vi "Main Control lasers.vi"() -> ()   [LabVIEW 2020]
uses:
  Control 1.ctl
  Control_states.ctl
  <vilib>/Analysis/baseanly.llb/Mean (DBL).vi
  <vilib>/ULx/Create Channel.llb/ULx Create Channel (AO-Voltage-Basic).vi
  <vilib>/ULx/Write.llb/ULx Write (Analog 1D DBL 1Chan NSamp).vi
  Global 1.vi
  <vilib>/ULx/Create Channel.llb/ULx Create Channel (DO-Digital Output).vi
  <vilib>/ULx/Write.llb/ULx Write (Digital Bool 1Line 1Point).vi
  <vilib>/ULx/Create Channel.llb/ULx Create Channel (AI-Voltage-Basic).vi
  <vilib>/ULx/Write.llb/ULx Write (Analog 1D DBL 1Chan 1Samp).vi
  <vilib>/ULx/Read.llb/ULx Read (Analog DBL 1Chan 1Samp).vi
  <vilib>/Analysis/NI_AALBase.lvlib
panel:
  in  "Tab Control 2":enum32{"Indicator"}(tab)
  out "Low Gain":dbl(graph)=1.648150384426117
  out "High Gain":dbl(graph)=143.05335879325867
  out "Data HG (mV)":dbl=143.05335879325867 format="%0.2f"
  out "Data LG (mV)":dbl=1.648150384426117 format="%0.2f"
  in  "SAVE":bool
  in  "stop":bool
  in  "Tab Control":T1(tab)
  in  "Frequency Selector (GHz)":i32(knob)=200 min=100 max=600 step=10 scale=100.0..600.0
  in  "Light":bool
  out "Stable output frequency":bool=TRUE
  in  "Stop Button":bool
  out "Current frequency (GHz)":dbl=200.0
  in  "Safety Switch":bool
  in  "Bias":bool
  in  "Sweep Activation":bool
  in  "Start (GHz)":dbl=100.0 min=100.0 max=600.0 step=10.0
  in  "Stop (GHz)":dbl=200.0 min=100.0 max=600.0 step=10.0
  in  "Time elapsed":T2
  in  "Time per point (ms)":u32=1000
  out "Current frequency monitor":dbl=200.0
  out "L2 ini":dbl=1.0008
  out "L1 ini":dbl=0.62712
  in  "contador":dbl=40.0
  in  "LD1 laser point":dbl=0.62712
  out "Current laser 1 (mA)":dbl=156.78
  out "Current laser 2 (mA)":dbl=250.2
  out "Laser":dbl=3.0
  out "String":string="estoy aqui"
  out "Signal OFF LG":dbl=-0.0037846416234970093 format="%0.2f"
  out "Signal ON LG":dbl=-0.005738005042076111 format="%0.2f"
  out "Difference LG":dbl=1.9533634185791016
  out "Difference HG":dbl=134.41584110259976
  out "Signal OFF HG":dbl=-3.054205846786499 format="%0.2f"
  out "Signal ON HG":dbl=-3.188621687889099 format="%0.2f"
  in  "Integration time (ms)":i32=20
  out "x+y":dbl=40.0
  in  "Ring":u16(ring) items=["600,93", "590,96", "580,92", "570,94", "561", "550,96", "541", "530,9", "520,97", "510,98", "500,96", "490,89", "480,99", "470,91", "460,92", "450,98", "440,98", "430,96", "420,95", "410,99", "400,92", "390,92", "381", "370,99", "360,92", "350,91", "340,97", "330,95", "320,99", "310,94", "300,94", "290,85", "280,97", "270,99", "260,9", "250,89", "240,92", "230,87", "220,83", "210,92", "200,98", "190,88", "180,96", "170,96", "160,95", "150,82", "140,96", "130,89", "120,87", "110,9", "100,95", "91", "80,85", "70,91", "60,99", "50,8", "40,88", "30,84", "20,78", "10,7"]
  out "OldVal":dbl
  out "corriente L1 2":dbl
  out "ok":bool
  in  "LD2 laser point":dbl=1.0008
  # "ON Sequence"
  # "OFF Sequence"
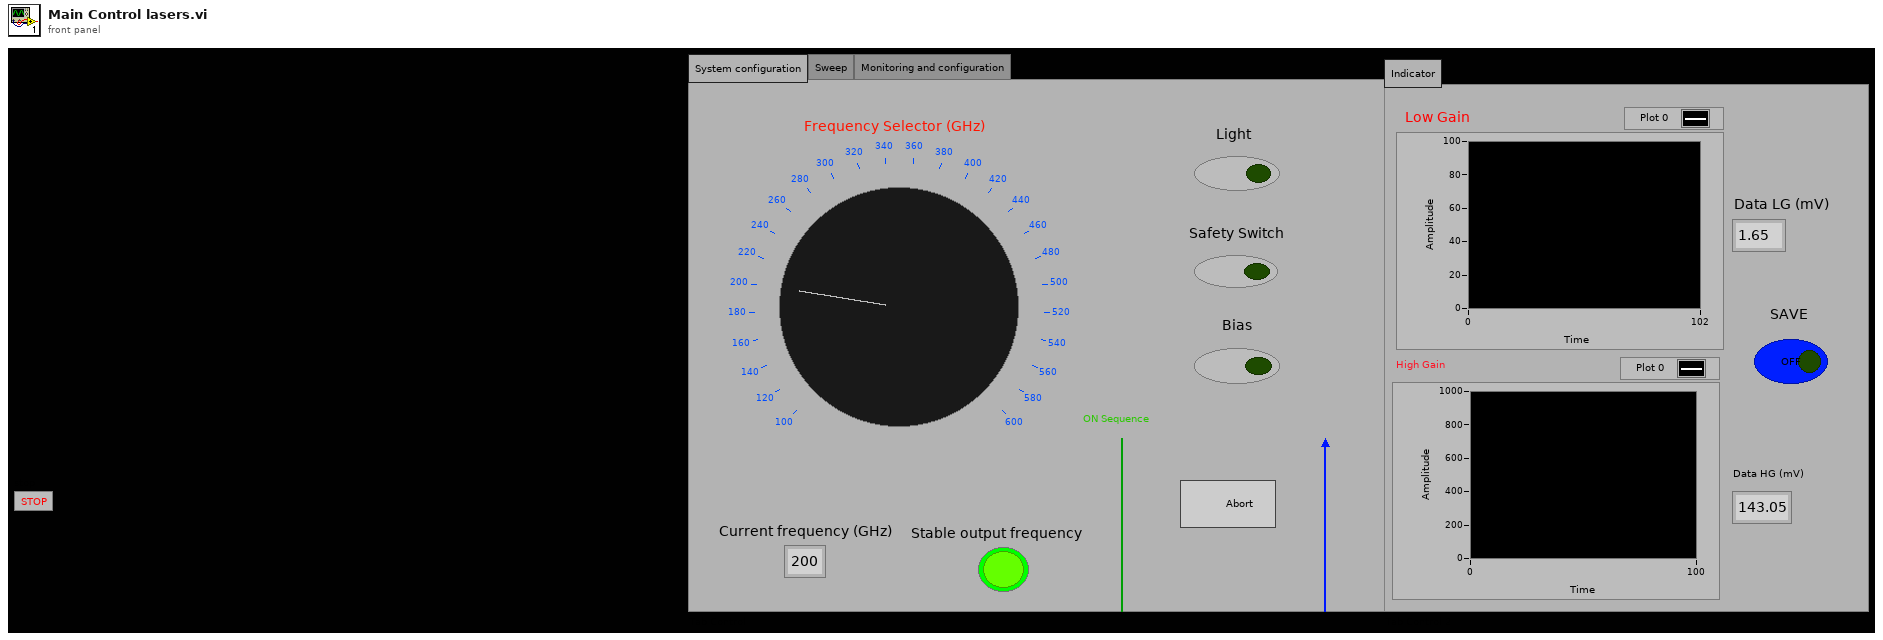
[diagram p1: front panel]
types:
  T1 = enum32{"System configuration", "Sweep", "Monitoring and configuration"}
  T2 = typedef "Control 1.ctl" = dbl
  T3 = typedef "Control_states.ctl" = enum16{"Rele", "Enable", "Corriente L2", "Sweep", "Atenuador", "Initializing", "Setting", "Modulacion", "Saving", "Control", "Closing"}
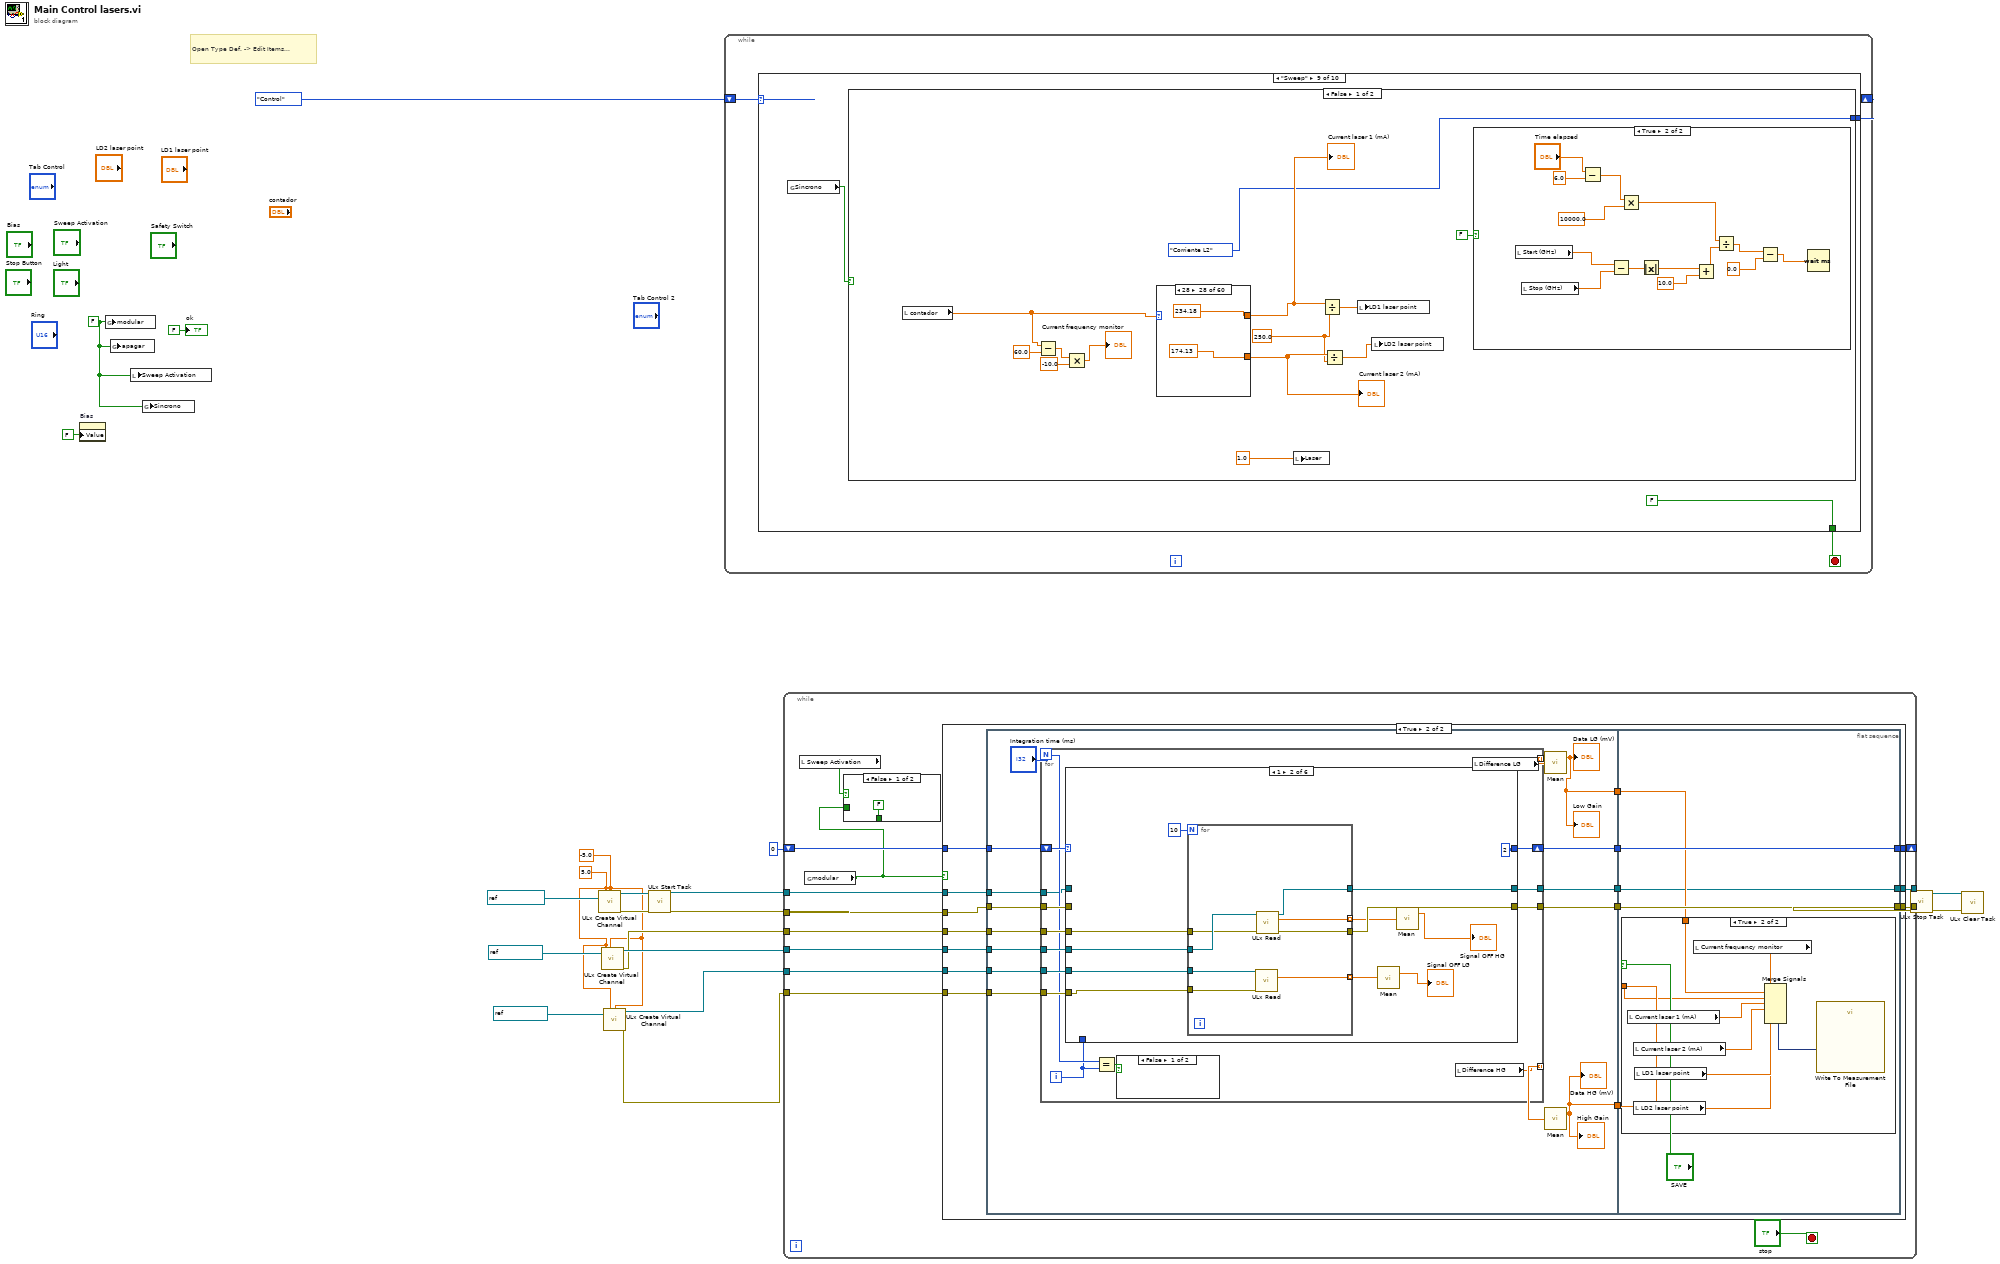
[diagram p0: block diagram]
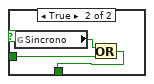
[diagram p2: hidden frame]
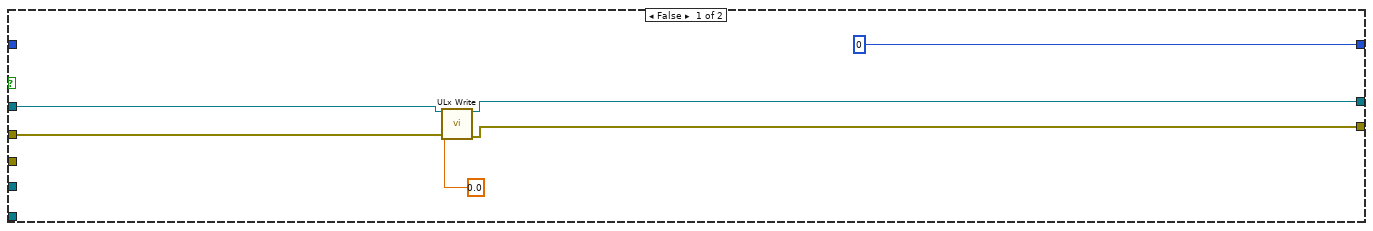
[diagram p3: hidden frame]
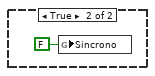
[diagram p4: hidden frame]
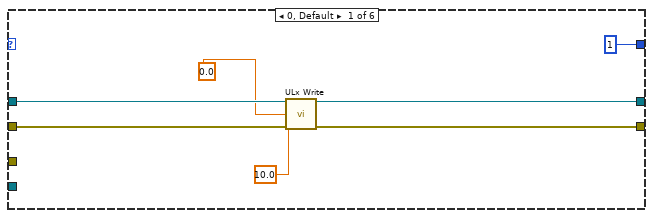
[diagram p5: hidden frame]
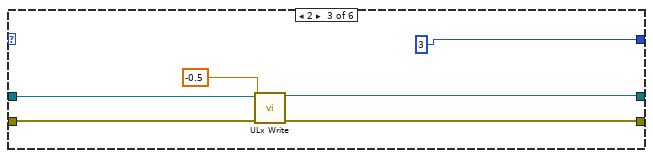
[diagram p6: hidden frame]
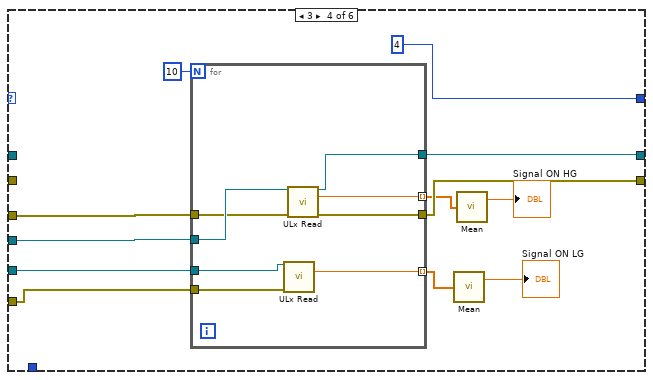
[diagram p7: hidden frame]
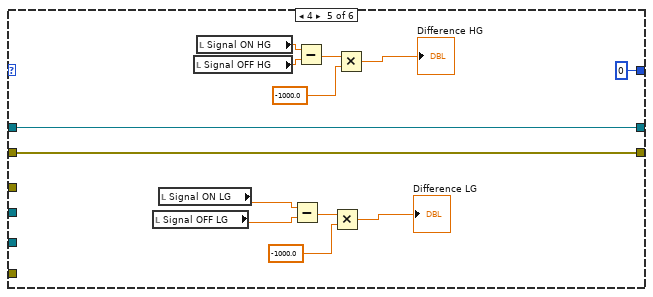
[diagram p8: hidden frame]
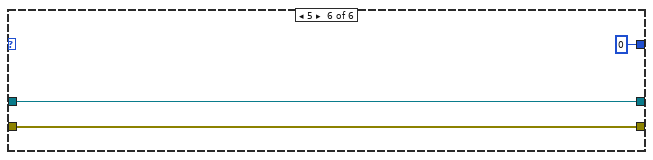
[diagram p9: hidden frame]
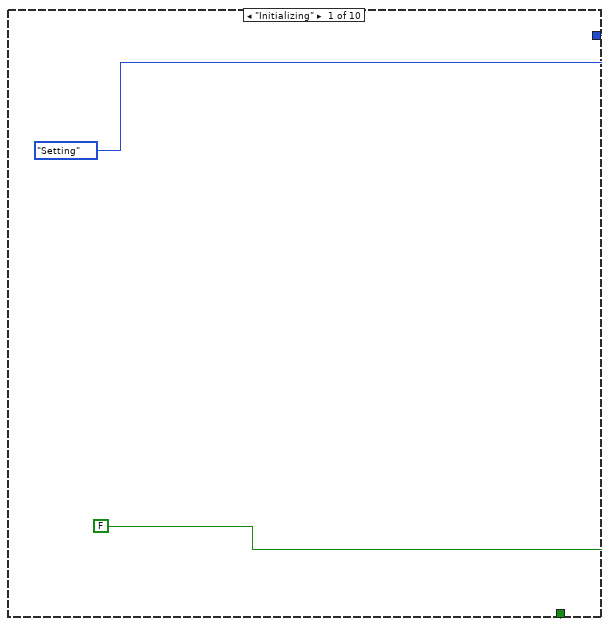
[diagram p11: hidden frame]
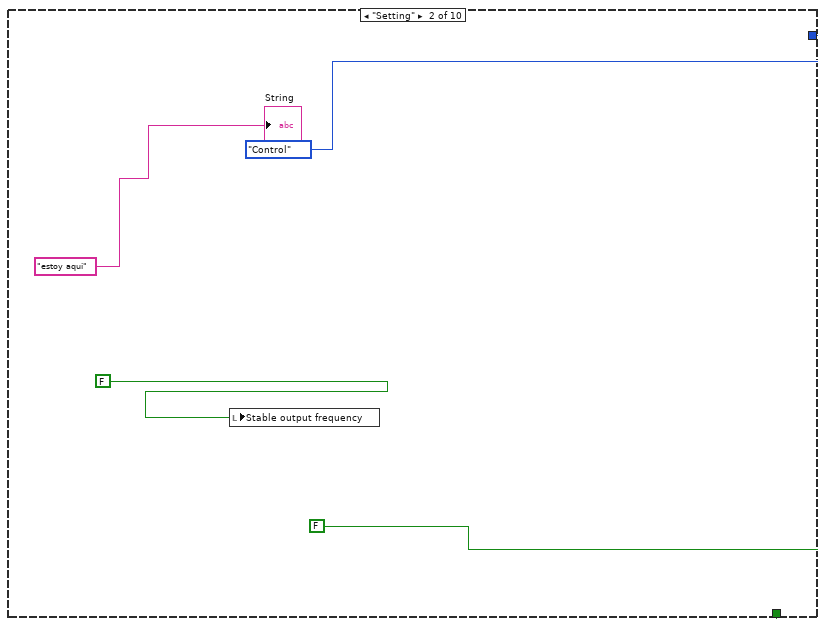
[diagram p12: hidden frame]
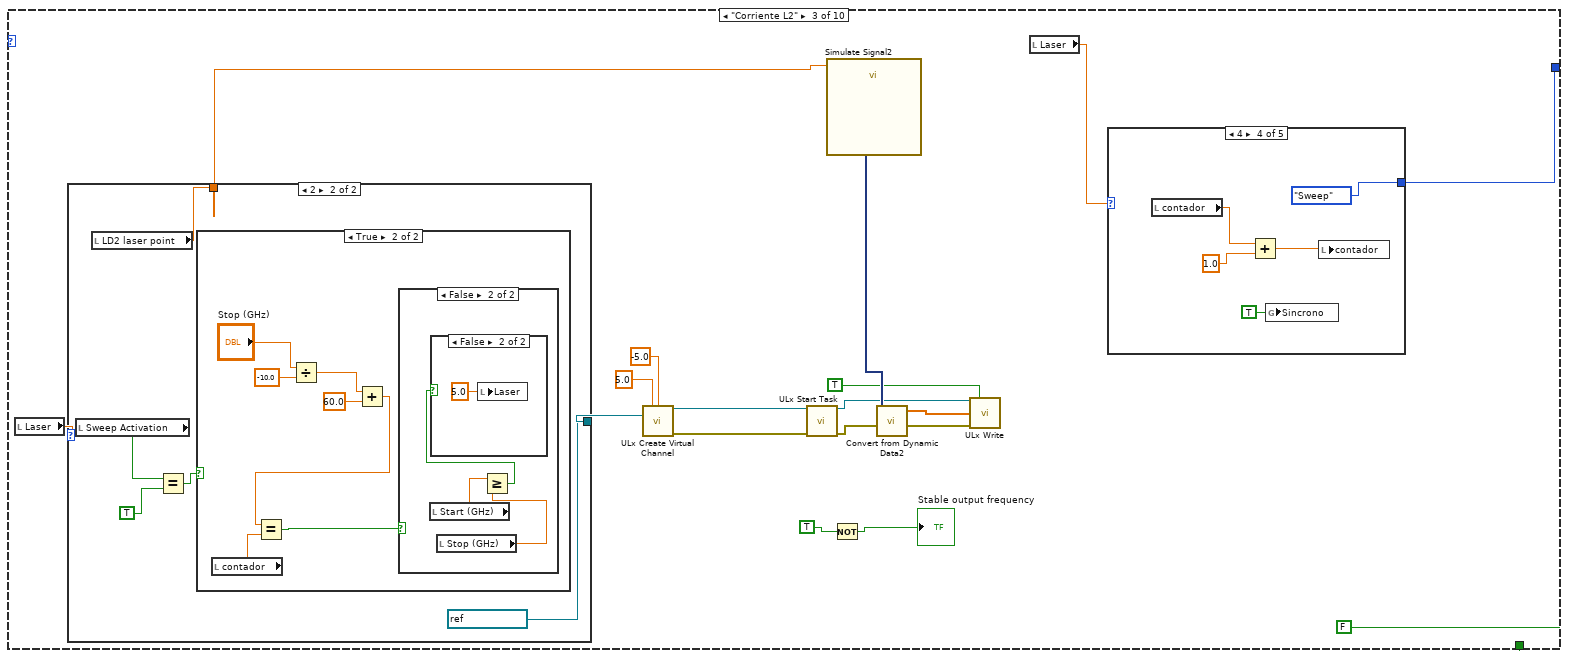
[diagram p13: hidden frame]
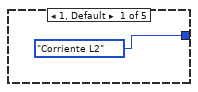
[diagram p14: hidden frame]
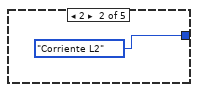
[diagram p15: hidden frame]
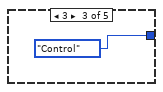
[diagram p16: hidden frame]
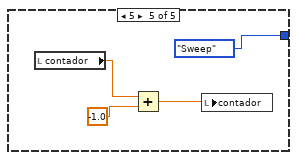
[diagram p17: hidden frame]
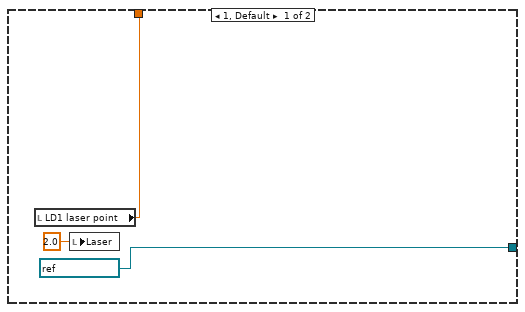
[diagram p18: hidden frame]
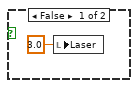
[diagram p19: hidden frame]
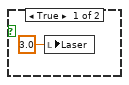
[diagram p20: hidden frame]
diagram:
  w2 = -5.0 ("minimum value")
  w3 = 5.0 ("maximum value")
  w6 = FALSE ("modular")
  # "Open Type Def. -> Edit Items..."
  n1 = property on="Bias" class="Bool (strict)"("Value"=FALSE ("Modular")) -> ()  [unwired: 2 in, 2 out]
  n2 = global write "Global 1.vi" "modular"(w6) -> ()
  n3 = global write "Global 1.vi" "apagar"(w6) -> ()
  n4 = local write "Sweep Activation"(w6) -> ()
  n5 = global write "Global 1.vi" "Sincrono"(w6) -> ()
  n6 = call-poly <vilib>:"ULx Create Virtual Channel.vi"("maximum value"=w3, "minimum value"=w2, "physical channels"=refnum<k21> "Dev0/Ao3") -> ("task out"=w19:refnum<k24>, "error out"=w18:errorcluster)  [unwired: 11 in]
  n7 = call-poly <vilib>:"ULx Create Virtual Channel.vi"("maximum value"=w3, "minimum value"=w2, "physical channels"=refnum<k21> "Dev0/Ai0") -> ("task out"=w12:refnum<k24>, "error out"=w11:errorcluster)  [unwired: 11 in]
  n8 = call-poly <vilib>:"ULx Create Virtual Channel.vi"("maximum value"=w3, "minimum value"=w2, "physical channels"=refnum<k21> "Dev0/Ai1") -> ("task out"=w1:refnum<k24>, "error out"=w4:errorcluster)  [unwired: 11 in]
  n9 = call <vilib>:"ULx Start Task.vi"("task in"=w19, "error in"=w18) -> ("task out"=w16:refnum<k24>, "error out"=w15:errorcluster)  [unwired: 12 in]
  n10 = while {
    shift-right: [w23] -> _
    shift-left: Control_states."Control" -> [w25]
    stop <- w24 stop-if-true
    n11 = case shown="\"Sweep\"" w25 {
      tunnel: [FALSE FALSE FALSE FALSE FALSE w87 FALSE FALSE FALSE FALSE] -> w24
      tunnel: [Control_states."Setting" Control_states."Control" w37 Control_states."Saving" Control_states."Control" Control_states."Closing" Control_states."Control" w99 w261 Control_states."Control"] -> w23
      frame "Initializing" {
      }
      frame "Setting" {
        n12 = local write "Stable output frequency"(FALSE ("L1 ok")) -> ()
        "String" <- "estoy aqui"
      }
      frame "Corriente L2" {
        n13 = local read "Laser"() -> (w39:dbl)
        n14 = case shown="2" w39 {
          tunnel: [refnum<k21> "Dev0/Ao0" ("physical channels") refnum<k21> "Dev0/Ao1" ("physical channels")] -> w46
          tunnel: [w62 w67] -> w38
          frame 1, Default {
            n15 = local read "LD1 laser point"() -> (w62:dbl)
            n16 = local write "Laser"(2.0 ("Laser")) -> ()
          }
          frame 2 {
            n17 = local read "Sweep Activation"() -> (w64:bool)
            n18 = local read "LD2 laser point"() -> (w67:dbl)
            n19 = Equal?(x=w64, y=TRUE) -> (x = y?=w66:bool)
            n20 = case shown="True" w66 {
              frame False {
                n21 = local write "Laser"(3.0 ("Laser")) -> ()
              }
              frame True {
                n22 = local read "contador"() -> (w75:dbl)
                n23 = Divide(x="Stop (GHz)", y=-10.0) -> (x/y=w73:dbl)
                n24 = Add(x=w73, y=60.0) -> (x+y=w70:dbl)
                n25 = Equal?(x=w70, y=w75) -> (x = y?=w76:bool)
                n26 = case shown="False" w76 {
                  frame True {
                    n27 = local write "Laser"(3.0 ("Laser")) -> ()
                  }
                  frame False {
                    n28 = local read "Start (GHz)"() -> (w80:dbl)
                    n29 = local read "Stop (GHz)"() -> (w79:dbl)
                    n30 = Greater Or Equal?(x=w80, y=w79) -> (x >= y?=w78:bool)
                    n31 = case shown="False" w78 {
                      frame True {
                        n32 = local write "Laser"(4.0 ("Laser")) -> ()
                      }
                      frame False {
                        n33 = local write "Laser"(5.0 ("Laser")) -> ()
                      }
                    }
                  }
                }
              }
            }
          }
        }
        n34 = call-poly <vilib>:"ULx Create Virtual Channel.vi"("maximum value"=5.0, "minimum value"=-5.0, "physical channels"=w46) -> ("task out"=w47:refnum<k24>, "error out"=w48:errorcluster)  [unwired: 11 in]
        n35 = call <vilib>:"ULx Start Task.vi"("task in"=w47, "error in"=w48) -> ("task out"=w42:refnum<k24>, "error out"=w41:errorcluster)  [unwired: 12 in]
        n36 = call "Simulate Signal2"("Offset"=w38) -> ("DC"=w45:dynamicdata)  [unwired: 13 in, 1 out]
        n37 = Not(x=TRUE) -> (.not. x?=→"Stable output frequency":bool)
        n38 = call "Convert from Dynamic Data2"("Dynamic Data Type"=w45) -> ("Array"=w44:dbl[])  [unwired: 3 in]
        n39 = call-poly <vilib>:"ULx Write.vi"("task in"=w42, "auto start"=TRUE, "data"=w44, "error in"=w41) -> ()  [unwired: 9 in, 3 out]
        n40 = local read "Laser"() -> (w36:dbl)
        n41 = case shown="4" w36 {
          tunnel: [Control_states."Corriente L2" Control_states."Corriente L2" Control_states."Control" Control_states."Sweep" Control_states."Sweep"] -> w37
          frame 1, Default {
          }
          frame 2 {
          }
          frame 3 {
          }
          frame 4 {
            n42 = local read "contador"() -> (w55:dbl)
            n43 = Add(x=w55, y=1.0) -> (x+y=w54:dbl)
            n44 = global write "Global 1.vi" "Sincrono"(TRUE ("Sincrono")) -> ()
            n45 = local write "contador"(w54) -> ()
          }
          frame 5 {
            n46 = local read "contador"() -> (w59:dbl)
            n47 = Add(x=w59, y=-1.0) -> (x+y=w58:dbl)
            n48 = local write "contador"(w58) -> ()
          }
        }
      }
      frame "Modulacion" {
      }
      frame "Saving" {
      }
      frame "Closing" {
        w87 = TRUE
        n49 = local write "Stable output frequency"(TRUE ("L1 ok")) -> ()
        n50 = global write "Global 1.vi" "apagar"(w87) -> ()
      }
      frame "Rele" {
        n51 = call-poly <vilib>:"ULx Create Virtual Channel.vi"("lines"=refnum<k21> "Dev0/AuxPort/Do9") -> ("task out"=w94:refnum<k24>, "error out"=w93:errorcluster)  [unwired: 13 in]
        n52 = local read "Safety Switch"() -> (w90:bool)
        n53 = call <vilib>:"ULx Start Task.vi"("task in"=w94, "error in"=w93) -> ("task out"=w92:refnum<k24>, "error out"=w91:errorcluster)  [unwired: 12 in]
        n54 = call-poly <vilib>:"ULx Write.vi"("task in"=w92, "data"=w90, "error in"=w91) -> ()  [unwired: 10 in, 3 out]
      }
      frame "Control", Default {
        n55 = event shown="[3] \"Frequency Selector (GHz)\": Value Change" {
          selector: _ -> [_ _ _ _ _ _ _ _]
          dyn-events: _ -> [_ _ _ _ _ _ _ _]
          timeout: 1 -> [_ _ _ _ _ _ _ _]
          tunnel: [Control_states."Control" Control_states."Atenuador" _ Control_states."Corriente L2" Control_states."Sweep" Control_states."Closing" Control_states."Enable" Control_states."Rele"] -> w99
          event Timeout {
            n56 = event-data() -> ()  [unwired: 1 in, 3 out]
            n57 = local read "LD2 laser point"() -> (→"L2 ini":dbl)
            n58 = local read "LD1 laser point"() -> (→"L1 ini":dbl)
            n59 = local write "Stable output frequency"(TRUE ("ok")) -> ()
          }
          event "LD1 laser point", "LD2 laser point": Value Change {
            n60 = event-data() -> ("OldVal"=w112:dbl)  [unwired: 1 in, 5 out]
            "OldVal" <- w112
            n61 = local read "LD1 laser point"() -> (w109:dbl)
            n62 = local read "L1 ini"() -> (w110:dbl)
            "corriente L1 2" <- w110
            n63 = Not Equal?(x=w110, y=w109) -> (x != y?=w108:bool)
            n64 = Equal?(x=w110, y=w112) -> (x = y?=w107:bool)
            n65 = And(x=w107, y=w108) -> (x .and. y?=w106:bool)
            n66 = case shown="False" w106 {
              tunnel: [2.0 ("Laser") 1.0 ("Laser")] -> w111
              frame False {
              }
              frame True {
              }
            }
            "Laser" <- w111
          }
          event "Bias": Value Change {
            n67 = event-data() -> ()  [unwired: 1 in, 6 out]
            n68 = global read "Global 1.vi" "modular"() -> (w116:bool)
            n69 = Not(x=w116) -> (.not. x?=w115:bool)
            n70 = global write "Global 1.vi" "modular"(w115) -> ()
          }
          event "Frequency Selector (GHz)": Value Change {
            w120 = 250.0 ("y")
            n71 = event-data() -> ()  [unwired: 1 in, 6 out]
            n72 = Divide(x="Frequency Selector (GHz)", y=-10.0) -> (x/y=w126:dbl)
            n73 = Add(x=w126, y=60.0) -> (x+y=w122:dbl)
            "x+y" <- w122
            n74 = case shown="9" w122 {
              tunnel: [52.69 57.03 59.36 63.7 66.7 69.7 73.37 76.71 82.05 86.05 90.39 94.39 97.73 102.4 107.07 112.07 116.08 121.42 126.75 131.43 136.1 141.77 146.77 152.11 157.45 162.79 168.46 174.13 180.13 186.14 192.48 198.48 204.16 210.83 216.83 223.51 229.85 236.85 243.19 250.2 257.54 264.21 271.55 278.56 286.23 293.57 300.91 308.58 316.26 323.93 331.94 339.94 347.95 355.96 364.3 372.31 380.65 388.99 397.33 46.68] -> w119
              tunnel: [398.66 392.99 386.98 381.31 375.31 369.3 363.3 357.29 351.62 345.61 339.61 333.6 327.27 321.26 315.25 309.25 302.91 296.91 290.9 284.56 278.22 272.22 265.88 259.54 253.2 246.86 240.52 234.18 227.84 221.5 215.17 208.83 202.15 195.82 189.14 182.8 176.13 169.79 163.12 156.78 150.44 143.77 137.43 130.76 124.42 118.08 111.41 105.07 98.73 92.39 86.39 80.05 74.04 68.04 62.03 56.02 50.35 44.68 39.01 404] -> w117
              frame 1, Default {
              }
              frame 2 {
              }
              frame 3 {
              }
              frame 4 {
              }
              frame 5 {
              }
              frame 6 {
              }
              frame 7 {
              }
              frame 8 {
              }
              frame 9 {
              }
              frame 10 {
              }
              frame 11 {
              }
              frame 12 {
              }
              frame 13 {
              }
              frame 14 {
              }
              frame 15 {
              }
              frame 16 {
              }
              frame 17 {
              }
              frame 18 {
              }
              frame 19 {
              }
              frame 20 {
              }
              frame 21 {
              }
              frame 22 {
              }
              frame 23 {
              }
              frame 24 {
              }
              frame 25 {
              }
              frame 26 {
              }
              frame 27 {
              }
              frame 28 {
              }
              frame 29 {
              }
              frame 30 {
              }
              frame 31 {
              }
              frame 32 {
              }
              frame 33 {
              }
              frame 34 {
              }
              frame 35 {
              }
              frame 36 {
              }
              frame 37 {
              }
              frame 38 {
              }
              frame 39 {
              }
              frame 40 {
              }
              frame 41 {
              }
              frame 42 {
              }
              frame 43 {
              }
              frame 44 {
              }
              frame 45 {
              }
              frame 46 {
              }
              frame 47 {
              }
              frame 48 {
              }
              frame 49 {
              }
              frame 50 {
              }
              frame 51 {
              }
              frame 52 {
              }
              frame 53 {
              }
              frame 54 {
              }
              frame 55 {
              }
              frame 56 {
              }
              frame 57 {
              }
              frame 58 {
              }
              frame 59 {
              }
              frame 0 {
              }
            }
            n75 = Divide(x=w117, y=w120) -> (x/y=w123:dbl)
            n76 = Divide(x=w119, y=w120) -> (x/y=w124:dbl)
            n77 = local write "Laser"(1.0 ("Laser")) -> ()
            n78 = local write "LD1 laser point"(w123) -> ()
            n79 = local write "LD2 laser point"(w124) -> ()
            "Current frequency (GHz)" <- "Frequency Selector (GHz)"
          }
          event "Sweep Activation": Value Change {
            n80 = event-data() -> ()  [unwired: 1 in, 6 out]
            n81 = Divide(x="Start (GHz)", y=-10.0) -> (x/y=w251:dbl)
            n82 = Add(x=w251, y=60.0) -> (x+y=w249:dbl)
            n83 = local write "contador"(w249) -> ()
          }
          event "Stop Button": Value Change {
            n84 = event-data() -> ()  [unwired: 1 in, 6 out]
            n85 = property on="Bias" class="Bool (strict)"("Value"=FALSE ("Modular")) -> ()  [unwired: 2 in, 2 out]
          }
          event "Light": Value Change {
            n86 = event-data() -> ()  [unwired: 1 in, 6 out]
          }
          event "Safety Switch": Value Change {
            n87 = event-data() -> ()  [unwired: 1 in, 6 out]
          }
        }
      }
      frame "Sweep" {
        n88 = global read "Global 1.vi" "Sincrono"() -> (w260:bool)
        n89 = case shown="False" w260 {
          tunnel: [Control_states."Corriente L2" Control_states."Control"] -> w261
          frame False {
            w269 = 250.0
            n90 = local read "contador"() -> (w265:dbl)
            n91 = Subtract(x=w265, y=60.0) -> (x-y=w264:dbl)
            n92 = Multiply(x=w264, y=-10.0) -> (x*y=→"Current frequency monitor":dbl)
            n93 = case shown="28" w265 {
              tunnel: [398.66 392.99 386.98 381.31 375.31 369.3 363.3 357.29 351.62 345.61 339.61 333.6 327.27 321.26 315.25 309.25 302.91 296.91 290.9 284.56 278.22 272.22 265.88 259.54 253.2 246.86 240.52 234.18 227.84 221.5 215.17 208.83 202.15 195.82 189.14 182.8 176.13 169.79 163.12 156.78 150.44 143.77 137.43 130.76 124.42 118.08 111.41 105.07 98.73 92.39 86.39 80.05 74.04 68.04 62.03 56.02 50.35 44.68 39.01 404.0] -> w271
              tunnel: [52.69 57.03 59.36 63.7 66.7 69.7 73.37 76.71 82.05 86.05 90.39 94.39 97.73 102.4 107.07 112.07 116.08 121.42 126.75 131.43 136.1 141.77 146.77 152.11 157.45 162.79 168.46 174.13 180.13 186.14 192.48 198.48 204.16 210.83 216.83 223.51 229.85 236.85 243.19 250.2 257.54 264.21 271.55 278.56 286.23 293.57 300.91 308.58 316.26 323.93 331.94 339.94 347.95 355.96 364.3 372.31 380.65 388.99 397.33 46.68] -> w272
              frame 1, Default {
              }
              frame 2 {
              }
              frame 3 {
              }
              frame 4 {
              }
              frame 5 {
              }
              frame 6 {
              }
              frame 7 {
              }
              frame 8 {
              }
              frame 9 {
              }
              frame 10 {
              }
              frame 11 {
              }
              frame 12 {
              }
              frame 13 {
              }
              frame 14 {
              }
              frame 15 {
              }
              frame 16 {
              }
              frame 17 {
              }
              frame 18 {
              }
              frame 19 {
              }
              frame 20 {
              }
              frame 21 {
              }
              frame 22 {
              }
              frame 23 {
              }
              frame 24 {
              }
              frame 25 {
              }
              frame 26 {
              }
              frame 27 {
              }
              frame 28 {
              }
              frame 29 {
              }
              frame 30 {
              }
              frame 31 {
              }
              frame 32 {
              }
              frame 33 {
              }
              frame 34 {
              }
              frame 35 {
              }
              frame 36 {
              }
              frame 37 {
              }
              frame 38 {
              }
              frame 39 {
              }
              frame 40 {
              }
              frame 41 {
              }
              frame 42 {
              }
              frame 43 {
              }
              frame 44 {
              }
              frame 45 {
              }
              frame 46 {
              }
              frame 47 {
              }
              frame 48 {
              }
              frame 49 {
              }
              frame 50 {
              }
              frame 51 {
              }
              frame 52 {
              }
              frame 53 {
              }
              frame 54 {
              }
              frame 55 {
              }
              frame 56 {
              }
              frame 57 {
              }
              frame 58 {
              }
              frame 59 {
              }
              frame 0 {
              }
            }
            "Current laser 1 (mA)" <- w271
            "Current laser 2 (mA)" <- w272
            n94 = local write "Laser"(1.0 ("Laser")) -> ()
            n95 = Divide(x=w271, y=w269) -> (x/y=w273:dbl)
            n96 = Divide(x=w272, y=w269) -> (x/y=w274:dbl)
            n97 = local write "LD1 laser point"(w273) -> ()
            n98 = local write "LD2 laser point"(w274) -> ()
            n99 = case shown="True" FALSE {
              frame False {
                n100 = Wait (ms)(milliseconds to wait="Time per point (ms)") -> ()  [unwired: 1 out]
              }
              frame True {
                n101 = local read "Start (GHz)"() -> (w279:dbl)
                n102 = local read "Stop (GHz)"() -> (w278:dbl)
                n103 = Subtract(x="Time elapsed", y=6.0) -> (x-y=w280:T2)
                n104 = Subtract(x=w279, y=w278) -> (x-y=w277:dbl)
                n105 = Multiply(x=w280, y=10000.0) -> (x*y=w289:T2)
                n106 = Absolute Value(x=w277) -> (abs(x)=w276:dbl)
                n107 = Add(x=w276, y=10.0) -> (x+y=w288:dbl)
                n108 = Divide(x=w289, y=w288) -> (x/y=w285:T2)
                n109 = Subtract(x=w285, y=0.0) -> (x-y=w284:T2)
                n110 = Wait (ms)(milliseconds to wait=w284) -> ()  [unwired: 1 out]
              }
            }
          }
          frame True {
          }
        }
      }
      frame "Enable" {
        n111 = call-poly <vilib>:"ULx Create Virtual Channel.vi"("lines"=refnum<k21> "Dev0/AuxPort/Do8") -> ("task out"=w416:refnum<k24>, "error out"=w417:errorcluster)  [unwired: 13 in]
        n112 = call <vilib>:"ULx Start Task.vi"("task in"=w416, "error in"=w417) -> ("task out"=w414:refnum<k24>, "error out"=w413:errorcluster)  [unwired: 12 in]
        n113 = local read "Light"() -> (w411:bool)
        n114 = Not(x=w411) -> (.not. x?=w412:bool)
        n115 = call-poly <vilib>:"ULx Write.vi"("task in"=w414, "data"=w412, "error in"=w413) -> ()  [unwired: 10 in, 3 out]
        n116 = case shown="True" w411 {
          frame False {
          }
          frame True {
            w420 = 200 ("Value (Signaling)")
            n117 = local write "Current frequency (GHz)"(w420) -> ()
            n118 = property on="Frequency Selector (GHz)" class="Knob (strict)"("Val(Sgnl)"=w420) -> ()  [unwired: 2 in, 2 out]
          }
        }
      }
    }
  }
  n119 = while {
    tunnel: w16 -> [w433]
    tunnel: w15 -> [w432]
    shift-right: [w430] -> _
    shift-left: 0 -> [w431]
    tunnel: w12 -> [w429]
    tunnel: w11 -> [w428]
    tunnel: [w427] -> w10
    tunnel: [w426] -> w9
    tunnel: w1 -> [w423]
    tunnel: w4 -> [w422]
    stop <- "stop" stop-if-true
    n120 = local read "Sweep Activation"() -> (w424:bool)
    n121 = global read "Global 1.vi" "modular"() -> (w421:bool)
    n122 = case shown="False" w424 {
      tunnel: w421 -> [_ w436]
      tunnel: [FALSE w435] -> _
      frame False {
      }
      frame True {
        n123 = global read "Global 1.vi" "Sincrono"() -> (w437:bool)
        n124 = Or(x=w437, y=w436) -> (x .or. y?=w435:bool)
      }
    }
    n125 = case shown="True" w421 {
      tunnel: w433 -> [w442 w450]
      tunnel: w432 -> [w441 w458]
      tunnel: w431 -> [_ w457]
      tunnel: [0 w456] -> w430
      tunnel: w429 -> [_ w455]
      tunnel: w428 -> [_ w454]
      tunnel: [w440 w449] -> w427
      tunnel: [w439 w453] -> w426
      tunnel: w423 -> [_ w452]
      tunnel: w422 -> [_ w451]
      frame False {
        n126 = call-poly <vilib>:"ULx Write.vi"("task in"=w442, "data"=0.0, "error in"=w441) -> ("task out"=w440:refnum<k24>, "error out"=w439:errorcluster)  [unwired: 10 in, 1 out]
      }
      frame True {
        n127 = flat-sequence {
          tunnel: w458 -> [w473]
          tunnel: w457 -> [w472]
          tunnel: w455 -> [w470]
          tunnel: w454 -> [w469]
          tunnel: w452 -> [w466]
          tunnel: w451 -> [w465]
          tunnel: w450 -> [w463]
          tunnel: [w471] -> w448
          tunnel: [w468] -> w447
          tunnel: [w462] -> w446
          tunnel: [w460] -> w445
          tunnel: [w459] -> w444
          tunnel: [w559] -> w449
          tunnel: [w563] -> w453
          tunnel: [w564] -> w456
          tunnel: w448 -> [w564]
          tunnel: w447 -> [w563]
          tunnel: w446 -> [w559]
          tunnel: w445 -> [w561]
          tunnel: w444 -> [w560]
          frame #0 {
            n128 = for {
              N: "Integration time (ms)" -> [w479]
              tunnel: w470 -> [w485]
              tunnel: w469 -> [w484]
              shift-right: [w486] -> w471
              shift-left: w472 -> [w487]
              tunnel: [w475] -> w464 mode=indexing
              tunnel: w466 -> [w481]
              tunnel: w465 -> [w480]
              tunnel: [w474] -> w461 mode=indexing
              tunnel: w463 -> [w478]
              tunnel: w473 -> [w488]
              tunnel: [w483] -> w468
              tunnel: [w477] -> w462
              i -> [w476]
              n129 = case shown="1" w487 {
                tunnel: w478 -> [w496 _ w522 _ w544 w557]
                tunnel: w488 -> [w495 _ w521 _ w543 w556]
                tunnel: [w493 w504 w520 w531 w544 w557] -> w477
                tunnel: [w492 w503 w519 w530 w543 w556] -> w483
                tunnel: [1 2 3 4 0 0] -> w486
                tunnel: w485 -> [_ w508 _ w532 _ _]
                tunnel: w484 -> [_ w507 _ w533 _ _]
                tunnel: w481 -> [_ w500 _ w526 _ _]
                tunnel: w480 -> [_ w499 _ w525 _ _]
                tunnel: w476 -> [_ _ _ _ _ _]
                frame 0, Default {
                  n130 = call-poly <vilib>:"ULx Write.vi"("task in"=w496, "data"=0.0 ("Min modulación"), "timeout"=10.0, "error in"=w495) -> ("task out"=w493:refnum<k24>, "error out"=w492:errorcluster)  [unwired: 9 in, 1 out]
                }
                frame 1 {
                  n131 = for {
                    N: 10 -> [_]
                    tunnel: w508 -> [w516]
                    tunnel: w507 -> [w515]
                    tunnel: [w514] -> w502 mode=indexing
                    tunnel: [w513] -> w504
                    tunnel: [w512] -> w503
                    tunnel: w500 -> [w511]
                    tunnel: w499 -> [w510]
                    tunnel: [w509] -> w498 mode=indexing
                    n132 = call-poly <vilib>:"ULx Read.vi"("task in"=w511, "error in"=w510) -> ("data"=w509:dbl)  [unwired: 11 in, 2 out]
                    n133 = call-poly <vilib>:"ULx Read.vi"("task in"=w516, "error in"=w515) -> ("task out"=w513:refnum<k24>, "data"=w514:dbl, "error out"=w512:errorcluster)  [unwired: 11 in]
                  }
                  n134 = call-poly <vilib>:"Mean.vi"("X"=w498) -> ("mean"=→"Signal OFF LG":dbl)  [unwired: 1 out]
                  n135 = call-poly <vilib>:"Mean.vi"("X"=w502) -> ("mean"=→"Signal OFF HG":dbl)  [unwired: 1 out]
                }
                frame 2 {
                  n136 = call-poly <vilib>:"ULx Write.vi"("task in"=w522, "data"=-0.5 ("Max modulación"), "error in"=w521) -> ("task out"=w520:refnum<k24>, "error out"=w519:errorcluster)  [unwired: 10 in, 1 out]
                }
                frame 3 {
                  n137 = for {
                    N: 10 -> [_]
                    tunnel: w532 -> [w542]
                    tunnel: w533 -> [w541]
                    tunnel: [w540] -> w528 mode=indexing
                    tunnel: [w539] -> w531
                    tunnel: [w538] -> w530
                    tunnel: w526 -> [w537]
                    tunnel: w525 -> [w536]
                    tunnel: [w535] -> w524 mode=indexing
                    n138 = call-poly <vilib>:"ULx Read.vi"("task in"=w537, "error in"=w536) -> ("data"=w535:dbl)  [unwired: 11 in, 2 out]
                    n139 = call-poly <vilib>:"ULx Read.vi"("task in"=w542, "error in"=w541) -> ("task out"=w539:refnum<k24>, "data"=w540:dbl, "error out"=w538:errorcluster)  [unwired: 11 in]
                  }
                  n140 = call-poly <vilib>:"Mean.vi"("X"=w524) -> ("mean"=→"Signal ON LG":dbl)  [unwired: 1 out]
                  n141 = call-poly <vilib>:"Mean.vi"("X"=w528) -> ("mean"=→"Signal ON HG":dbl)  [unwired: 1 out]
                }
                frame 4 {
                  n142 = local read "Signal OFF LG"() -> (w547:dbl)
                  n143 = local read "Signal ON LG"() -> (w548:dbl)
                  n144 = local read "Signal OFF HG"() -> (w554:dbl)
                  n145 = local read "Signal ON HG"() -> (w555:dbl)
                  n146 = Subtract(x=w548, y=w547) -> (x-y=w550:dbl)
                  n147 = Subtract(x=w555, y=w554) -> (x-y=w553:dbl)
                  n148 = Multiply(x=w550, y=-1000.0) -> (x*y=→"Difference LG":dbl)
                  n149 = Multiply(x=w553, y=-1000.0) -> (x*y=→"Difference HG":dbl)
                }
                frame 5 {
                }
              }
              n150 = Equal?(x=w479, y=w476) -> (x = y?=w482:bool)
              n151 = case shown="False" w482 {
                frame False {
                }
                frame True {
                  n152 = global write "Global 1.vi" "Sincrono"(FALSE ("Sincrono")) -> ()
                }
              }
              n153 = local read "Difference HG"() -> (w474:dbl)
              n154 = local read "Difference LG"() -> (w475:dbl)
            }
            n155 = call-poly <vilib>:"Mean.vi"("X"=w464) -> ("mean"=w460:dbl)  [unwired: 1 out]
            "Data LG (mV)" <- w460
            "Low Gain" <- w460
            n156 = call-poly <vilib>:"Mean.vi"("X"=w461) -> ("mean"=w459:dbl)  [unwired: 1 out]
            "Data HG (mV)" <- w459
            "High Gain" <- w459
          }
          frame #1 {
            n157 = case shown="True" "SAVE" {
              tunnel: w561 -> [_ w571]
              tunnel: w560 -> [_ w569]
              frame False {
              }
              frame True {
                n158 = local read "Current laser 1 (mA)"() -> (w565:dbl)
                n159 = local read "Current laser 2 (mA)"() -> (w568:dbl)
                n160 = local read "LD2 laser point"() -> (w566:dbl)
                n161 = local read "LD1 laser point"() -> (w567:dbl)
                n162 = local read "Current frequency monitor"() -> (w572:dbl)
                n163 = Merge Signals "Merge Signals"(w572, w571, w569, w565, w568, w567, w566) -> (w570:dynamicdata)
                n164 = call "Write To Measurement File"("Signals"=w570) -> ()  [unwired: 16 in, 3 out]
              }
            }
          }
        }
      }
    }
  }
  n165 = call <vilib>:"ULx Stop Task.vi"("error in"=w9, "task in"=w10) -> ("error out"=w7:errorcluster, "task out"=w8:refnum<k24>)  [unwired: 8 in]
  n166 = call <vilib>:"ULx Clear Task.vi"("task in"=w8, "error in"=w7) -> ()  [unwired: 13 in, 1 out]
  "ok" <- FALSE ("ok")
